vi "Set measurementservice_MUXCloseSessionRequest.vi"(7 "Complete Call (T)":bool=TRUE, 8 "error in (no error)":errorcluster, 10 "Message Data":T1, 11 "gRPCid":T2) -> (0 "error out":errorcluster)   [LabVIEW 2019, in "ctet_mux.lvlib" / "ctet_mux.lvclass"]
uses:
  ctet_mux.lvclass
  gRPC lvSupport/Server API/typeDefs/grpcId.ctl
  measurementservice_MUXCloseSessionRequest_Data.ctl
  dcc74a39-081a-4bdd-860b-8ed792803c96.vi
  gRPC lvSupport/Server API/Server/Get Server DLL Path.vi
  <vilib>/Utility/error.llb/Error Cluster From Error Code.vi
  gRPC lvSupport/gprc-lvsupport.lvlib
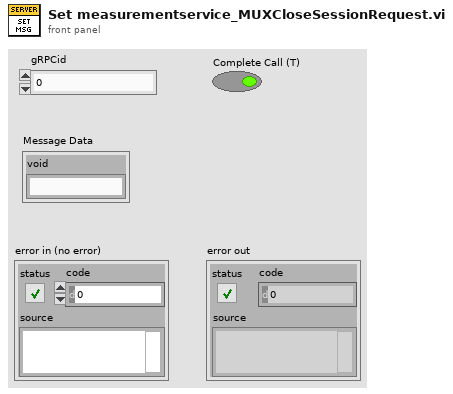
[diagram p1: front panel]
types:
  T1 = typedef "ctet_mux.lvlib/ctet_mux.lvclass/measurementservice_MUXCloseSessionRequest_Data.ctl" = cluster{"void":string}
  T2 = typedef "ctet_mux.lvlib/gprc-lvsupport.lvlib/grpcId.ctl" = u64
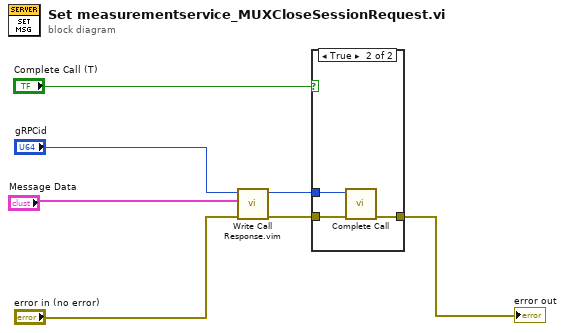
[diagram p0: block diagram]
diagram:
  n1 = call "Write Call Response.vim"("error in (no error)"="error in (no error)", "Response Data"="Message Data", "gRPCid in"="gRPCid") -> ("error out"=w4:errorcluster, "gRPCid"=w5:T2)  [unwired: 7 in]
  n2 = case shown="True" "Complete Call (T)" {
    tunnel: [w8 w11] -> w7
    tunnel: w5 -> [_ w10]
    tunnel: w4 -> [w8 w9]
    frame False {
    }
    frame True {
      n3 = call "Complete Call.vi"("gRPCid"=w10, "error in (no error)"=w9) -> ("error out"=w11:errorcluster)  [unwired: 8 in]
    }
  }
  "error out" <- w7
